vi "ApplyCorrection.vi"(9 "Pixel calibration":T1, 10 "Buffer Image":T2, 11 "Camera Image":T2) -> (3 "Refnum out":T2)   [LabVIEW 2011]
uses:
  <vilib>/vision/Image Controls.llb/IMAQ Image.ctl
  Camera/PixelCalibrationDataType.ctl
  <vilib>/vision/NI_Vision_Development_Module.lvlib
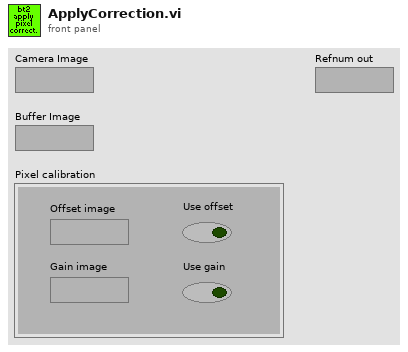
[diagram p1: front panel]
types:
  T1 = typedef "PixelCalibrationDataType.ctl" = cluster{"Offset image":T2, "Gain image":T2, "Use offset":bool, "Use gain":bool}
  T2 = typedef "IMAQ Image.ctl" = refnum<image>
  T3 = typedef "Image Type" = u32
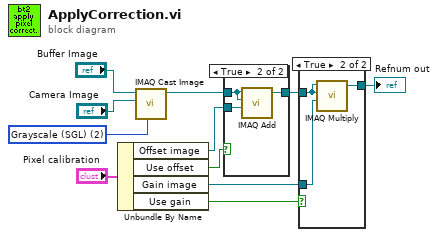
[diagram p0: block diagram]
diagram:
  w10 = T3 2 items=["Grayscale (U8)", "Grayscale (I16)", "Grayscale (SGL)", "Complex (CSG)", "RGB (U32)", "HSL (U32)", "RGB (U64)", "Grayscale (U16)"] ("Image Type")
  n1 = Unbundle By Name("Pixel calibration") -> ("Offset image"=w7:T2, "Use offset"=w5:bool, "Gain image"=w1:T2, "Use gain"=w4:bool)
  n2 = call "IMAQ Cast Image"("Image Type"=w10, "Image Dst"="Camera Image", "Image Src"="Buffer Image") -> ("Image Dst Out"=w11:T2)  [unwired: 7 in, 1 out]
  n3 = case shown="True" w5 {
    tunnel: w11 -> [w12 w15]
    tunnel: w7 -> [_ w14]
    tunnel: [w12 w13] -> w3
    frame False {
    }
    frame True {
      n4 = call "IMAQ Add"("Image Src A"=w15, "Image Dst"=w15, "Image Src B"=w14) -> ("Image Dst Out"=w13:T2)  [unwired: 4 in, 1 out]
    }
  }
  n5 = case shown="True" w4 {
    tunnel: w3 -> [w16 w19]
    tunnel: [w16 w17] -> w2
    tunnel: w1 -> [_ w18]
    frame False {
    }
    frame True {
      n6 = call "IMAQ Multiply"("Image Src A"=w19, "Image Dst"=w19, "Image Src B"=w18) -> ("Image Dst Out"=w17:T2)  [unwired: 4 in, 1 out]
    }
  }
  "Refnum out" <- w2
